vi "AccelCalc_subsubvi.vi"(6 "DeltaT":dbl, 7 "yk":dbl, 8 "k":dbl, 9 "m":dbl, 10 "b":dbl, 11 "xk":dbl) -> (1 "Accel 2":dbl, 3 "Accel":dbl)   [LabVIEW 2019]
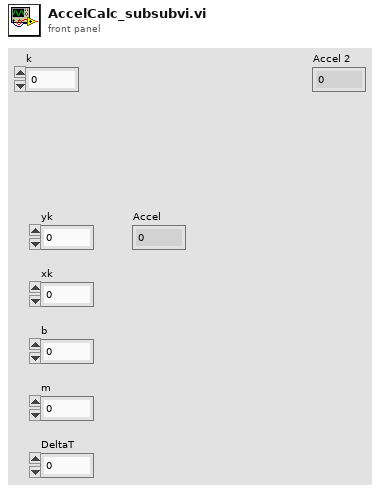
[diagram p1: front panel]
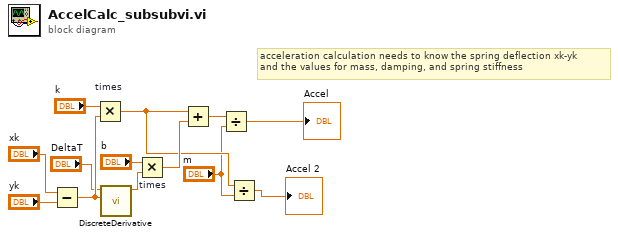
[diagram p0: block diagram]
diagram:
  # "acceleration calculation needs to know the spring deflection xk-yk\nand the values for mass, damping, and spring stiffness"
  n1 = Subtract(x="xk", y="yk") -> (x-y=w10:dbl)
  n2 = Multiply "times"(x="k", y=w10) -> (x*y=w3:dbl)
  n3 = call "DiscreteDerivative.vi"("data"=w10, "deltaT"="DeltaT") -> ("(data-data_old)/delT"=w11:dbl)  [unwired: 9 in]
  n4 = Multiply "times"(x="b", y=w11) -> (x*y=w12:dbl)
  n5 = Add(x=w3, y=w12) -> (x+y=w13:dbl)
  n6 = Divide(x=w13, y="m") -> (x/y=→"Accel":dbl)
  n7 = Divide(x=w3, y="m") -> (x/y=→"Accel 2":dbl)
